vi "SVC.vi"(8 "error in":errorcluster) -> (0 "error out":errorcluster, 3 "out":refnum<class "SVC.lvclass">)   [LabVIEW 2020]
doc: "C-Support Vector Classification.\n\n The implementation is based on libsvm. The fit time scales at least\n quadratically with the number of samples and may be impractical\n beyond tens of thousands of samples. For large datasets\n consider using :class:`~sklearn.svm.LinearSVC` or\n :class:`~sklearn.linear_model.SGDClassifier` instead, possibly after a\n :class:`~sklearn.kernel_approximation.Nystroem` transformer.\n\n The multiclass support is handled according to a one-vs-one scheme.\n\n For details on the precise mathematical formulation of the provided\n kernel functions and how `gamma`, `coef0` and `degree` affect each\n other, see the corresponding section in the narrative documentation:\n :ref:`svm_kernels`.\n\n Read more in the :ref:`User Guide <svm_classification>`.\n\n Parameters\n ----------\n C : float, default=1.0\n Regularization parameter. The strength of the regularization is\n inversely proportional to C. Must be strictly positive. The penalty\n is a squared l2 penalty.\n\n kernel : {'linear', 'poly', 'rbf', 'sigmoid', 'precomputed'}, default='rbf'\n Specifies the kernel type to be used in the algorithm.\n It must be one of 'linear', 'poly', 'rbf', 'sigmoid', 'precomputed' or\n a callable.\n If none is given, 'rbf' will be used. If a callable is given it is\n used to pre-compute the kernel matrix from data matrices; that matrix\n should be an array of shape ``(n_samples, n_samples)``.\n\n degree : int, default=3\n Degree of the polynomial kernel function ('poly').\n Ignored by all other kernels.\n\n gamma : {'scale', 'auto'} or float, default='scale'\n Kernel coefficient for 'rbf', 'poly' and 'sigmoid'.\n\n - if ``gamma='scale'`` (default) is passed then it uses\n 1 / (n_features * X.var()) as value of gamma,\n - if 'auto', uses 1 / n_features.\n\n .. versionchanged:: 0.22\n The default value of ``gamma`` changed from 'auto' to 'scale'.\n\n coef0 : float, default=0.0\n Independent term in kernel function.\n It is only significant in 'poly' and 'sigmoid'.\n\n shrinking : bool, default=True\n Whether to use the shrinking heuristic.\n See the :ref:`User Guide <shrinking_svm>`.\n\n probability : bool, default=False\n Whether to enable probability estimates. This must be enabled prior\n to calling `fit`, will slow down that method as it internally uses\n 5-fold cross-validation, and `predict_proba` may be inconsistent with\n `predict`. Read more in the :ref:`User Guide <scores_probabilities>`.\n\n tol : float, default=1e-3\n Tolerance for stopping criterion.\n\n cache_size : float, default=200\n Specify the size of the kernel cache (in MB).\n\n class_weight : dict or 'balanced', default=None\n Set the parameter C of class i to class_weight[i]*C for\n SVC. If not given, all classes are supposed to have\n weight one.\n The \"balanced\" mode uses the values of y to automatically adjust\n weights inversely proportional to class frequencies in the input data\n as ``n_samples / (n_classes * np.bincount(y))``\n\n verbose : bool, default=False\n Enable verbose output. Note that this setting takes advantage of a\n per-process runtime setting in libsvm that, if enabled, may not work\n properly in a multithreaded context.\n\n max_iter : int, default=-1\n Hard limit on iterations within solver, or -1 for no limit.\n\n decision_function_shape : {'ovo', 'ovr'}, default='ovr'\n Whether to return a one-vs-rest ('ovr') decision function of shape\n (n_samples, n_classes) as all other classifiers, or the original\n one-vs-one ('ovo') decision function of libsvm which has shape\n (n_samples, n_classes * (n_classes - 1) / 2). However, one-vs-one\n ('ovo') is always used as multi-class strategy. The parameter is\n ignored for binary classification.\n\n .. versionchanged:: 0.19\n decision_function_shape is 'ovr' by default.\n\n .. versionadded:: 0.17\n *decision_function_shape='ovr'* is recommended.\n\n .. versionchanged:: 0.17\n Deprecated *decision_function_shape='ovo' and None*.\n\n break_ties : bool, default=False\n If true, ``decision_function_shape='ovr'``, and number of classes > 2,\n :term:`predict` will break ties according to the confidence values of\n :term:`decision_function`; otherwise the first class among the tied\n classes is returned. Please note that breaking ties comes at a\n relatively high computational cost compared to a simple predict.\n\n .. versionadded:: 0.22\n\n random_state : int, RandomState instance or None, default=None\n Controls the pseudo random number generation for shuffling the data for\n probability estimates. Ignored when `probability` is False.\n Pass an int for reproducible output across multiple function calls.\n See :term:`Glossary <random_state>`.\n\n Attributes\n ----------\n class_weight_ : ndarray of shape (n_classes,)\n Multipliers of parameter C for each class.\n Computed based on the ``class_weight`` parameter.\n\n classes_ : ndarray of shape (n_classes,)\n The classes labels.\n\n coef_ : ndarray of shape (n_classes * (n_classes - 1) / 2, n_features)\n Weights assigned to the features (coefficients in the primal\n problem). This is only available in the case of a linear kernel.\n\n `coef_` is a readonly property derived from `dual_coef_` and\n `support_vectors_`.\n\n dual_coef_ : ndarray of shape (n_classes -1, n_SV)\n Dual coefficients of the support vector in the decision\n function (see :ref:`sgd_mathematical_formulation`), multiplied by\n their targets.\n For multiclass, coefficient for all 1-vs-1 classifiers.\n The layout of the coefficients in the multiclass case is somewhat\n non-trivial. See the :ref:`multi-class section of the User Guide\n <svm_multi_class>` for details.\n\n fit_status_ : int\n 0 if correctly fitted, 1 otherwise (will raise warning)\n\n intercept_ : ndarray of shape (n_classes * (n_classes - 1) / 2,)\n Constants in decision function.\n\n support_ : ndarray of shape (n_SV)\n Indices of support vectors.\n\n support_vectors_ : ndarray of shape (n_SV, n_features)\n Support vectors.\n\n n_support_ : ndarray of shape (n_classes,), dtype=int32\n Number of support vectors for each class.\n\n probA_ : ndarray of shape (n_classes * (n_classes - 1) / 2)\n probB_ : ndarray of shape (n_classes * (n_classes - 1) / 2)\n If `probability=True`, it corresponds to the parameters learned in\n Platt scaling to produce probability estimates from decision values.\n If `probability=False`, it's an empty array. Platt scaling uses the\n logistic function\n ``1 / (1 + exp(decision_value * probA_ + probB_))``\n where ``probA_`` and ``probB_`` are learned from the dataset [2]_. For\n more information on the multiclass case and training procedure see\n section 8 of [1]_.\n\n shape_fit_ : tuple of int of shape (n_dimensions_of_X,)\n Array dimensions of training vector ``X``.\n\n \nAvailable methods:\nFit\nPredict\nScore\nGet Attributes\nGet Params\nSet Params"
uses:
  SVC.lvclass
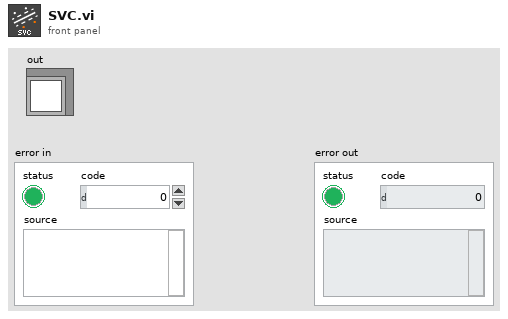
[diagram p1: front panel]
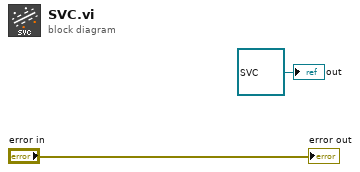
[diagram p0: block diagram]
diagram:
  "out" <- refnum<class "SVC.lvclass"> refnum ("model")
  "error out" <- "error in"
